vi "Set Material Velocity.vi"(7 "Micropulse # In":i32, 8 "error in (no error)":errorcluster, 10 "Material Velocity (m/s)":dbl=1.0) -> (0 "error out":errorcluster, 5 "Micropulse # Out":i32)   [LabVIEW 2026, in "MicroPulse_Driver.lvlib"]
doc: "Sets the material velocity which is used by the time to distance conversion routines"
uses:
  MicroPulse_Driver.lvlib
  Private/MP-Registry Action-Enum.ctl
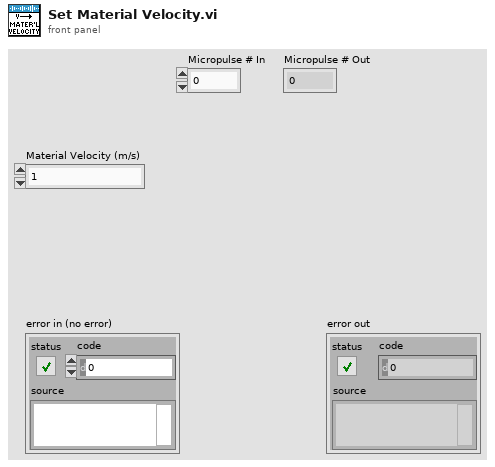
[diagram p1: front panel]
types:
  T1 = typedef "MicroPulse_Driver.lvlib/MP-Registry Action-Enum.ctl" = enum16{"Read", "Add Test", "Add Command", "Add Gate Command", "Add Encoder Command", "Clear Command  List", "Set Registry", "Set System Details", "Set DOF", "Set Velocity", "Disable Asynch Reads", "Enable Asynch Reads", "Add Connection", "Disconnect", "Shutdown"}
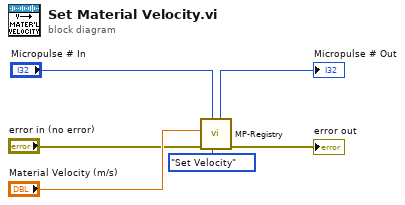
[diagram p0: block diagram]
diagram:
  n1 = call "MP-Registry.vi"("Action"=MP-Registry_Action-Enum."Set Velocity", "Micropulse # In"="Micropulse # In", "error in (no error)"="error in (no error)", "Data in"="Material Velocity (m/s)") -> ("error out"=→"error out":errorcluster, "Micropulse # Out"=→"Micropulse # Out":i32)  [unwired: 4 in, 2 out]
